vi "3- image processing.vi"() -> ()   [LabVIEW 2016]
uses:
  <vilib>/Instr/_visa.llb/VISA Configure Serial Port (Instr).vi
  <vilib>/vision/NI_Vision_Development_Module.lvlib
panel:
  out "decimal integer string 2":string
  out "decimal integer string":string
  in  "VISA resource name 4":refnum<visa-resource-name>
  out "return count 2":u32
  out "red":dbl
  out "green":dbl
  in  "VISA resource name 3":refnum<visa-resource-name>
  out "return count":u32
  out "green":bool
  out "red":bool
  out "Color Spectrum":dbl[](array[numeric]) format="%.2f"
  in  "Stop (F)":bool
  out "Image Out":T1(plugin-control)
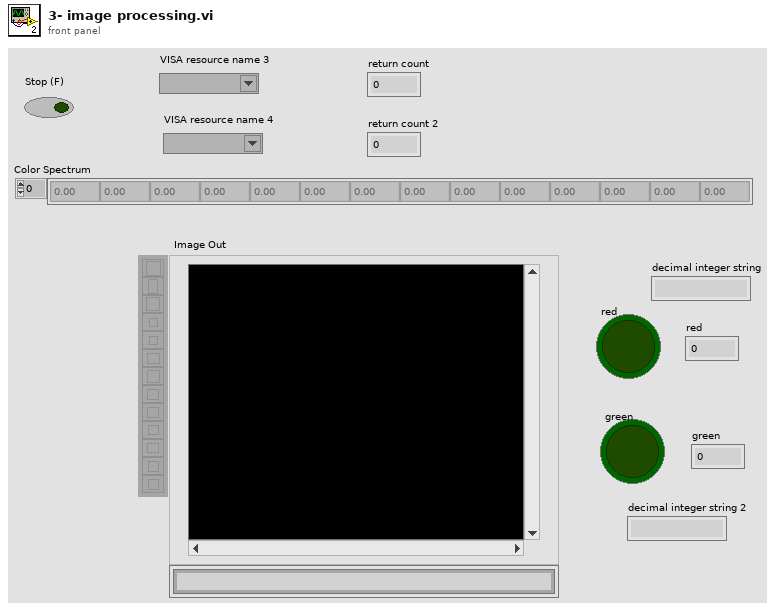
[diagram p1: front panel]
types:
  T1 = typedef "IMAQ Image.ctl" = refnum<image>
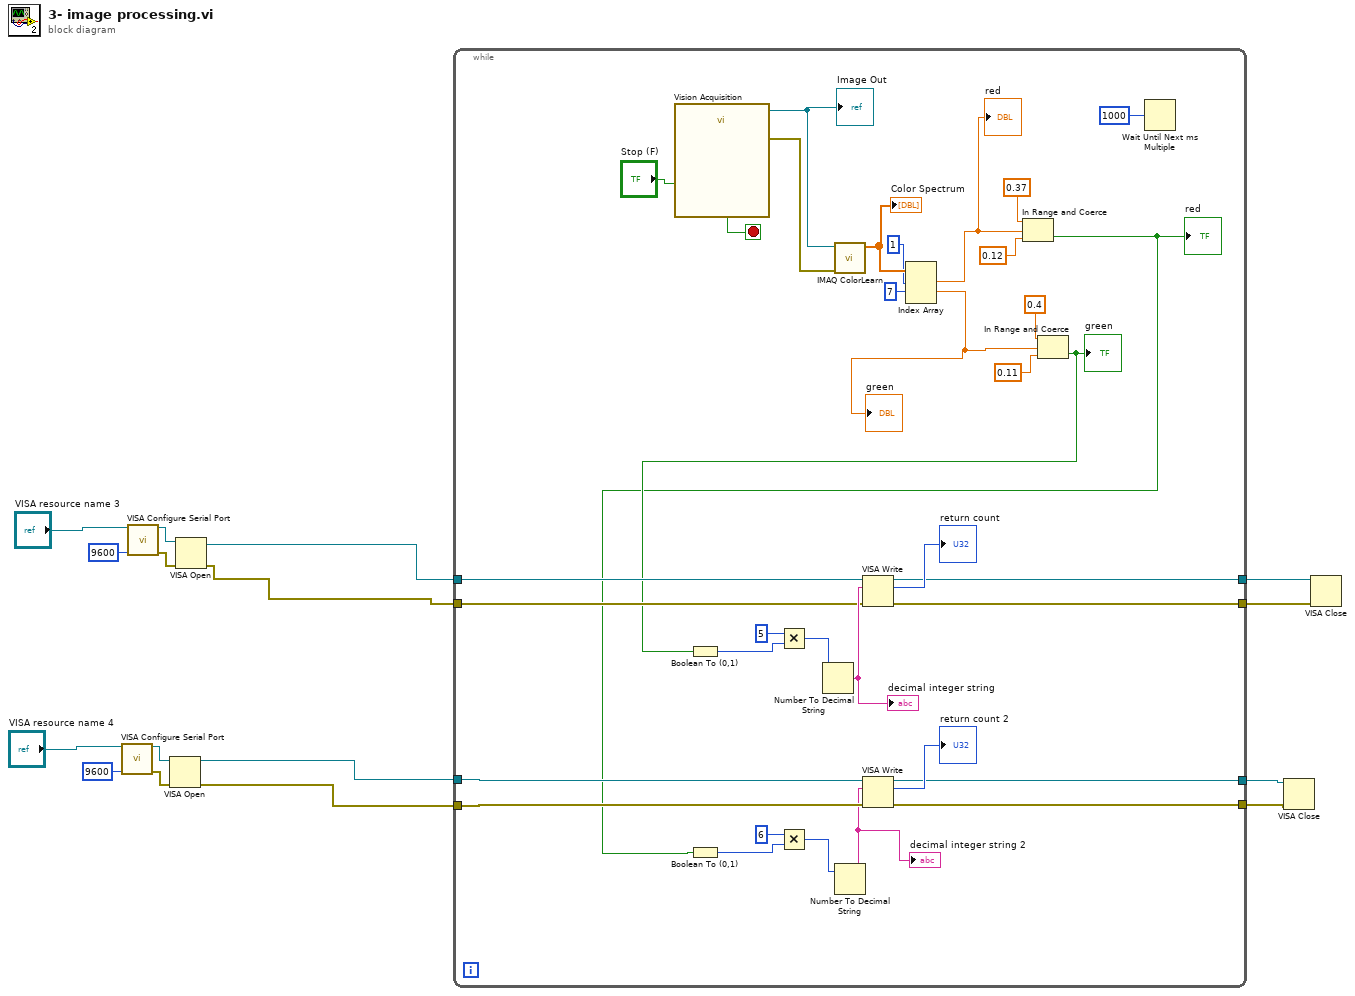
[diagram p0: block diagram]
diagram:
  n1 = call-poly "VISA Configure Serial Port"("VISA resource name"="VISA resource name 4", "baud rate (9600)"=u32 9600) -> ("VISA resource name out"=w6:refnum<visa-resource-name>, "error out"=w5:errorcluster)  [unwired: 12 in]
  n2 = call-poly "VISA Configure Serial Port"("VISA resource name"="VISA resource name 3", "baud rate (9600)"=u32 9600) -> ("VISA resource name out"=w14:refnum<visa-resource-name>, "error out"=w13:errorcluster)  [unwired: 12 in]
  n3 = VISA Open(error in (no error)=w5, VISA resource name=w6) -> (VISA resource name=w4:refnum<visa-resource-name>, error out=w3:errorcluster)  [unwired: 3 in]
  n4 = VISA Open(error in (no error)=w13, VISA resource name=w14) -> (VISA resource name=w10:refnum<visa-resource-name>, error out=w9:errorcluster)  [unwired: 3 in]
  n5 = while {
    tunnel: [w34] -> w12
    tunnel: [w33] -> w11
    tunnel: w10 -> [w32]
    tunnel: w9 -> [w31]
    tunnel: w4 -> [w23]
    tunnel: w3 -> [w22]
    tunnel: [w21] -> w2
    tunnel: [w20] -> w1
    stop <- w49 stop-if-true
    n6 = call "Vision Acquisition"("Stop (F)"="Stop (F)") -> ("Image Out"=w48:T1, "Stopped"=w49:bool, "error out"=w40:errorcluster)  [unwired: 24 in]
    "Image Out" <- w48
    n7 = call "IMAQ ColorLearn"("Image"=w48, "error in (no error)"=w40) -> ("Color Spectrum"=w47:dbl[])  [unwired: 6 in, 1 out]
    "Color Spectrum" <- w47
    n8 = Index Array(array=w47, index #1=1 ("index"), index #2=7 ("index")) -> (element #1=w18:dbl, element #2=w28:dbl)  [unwired: 1 in, 1 out]
    "green" <- w28
    "red" <- w18
    n9 = In Range and Coerce(upper limit=0.37, x=w18, lower limit=0.12) -> (In Range?=w19:bool)  [unwired: 1 out]
    "red" <- w19
    n10 = Boolean To (0,1)(Boolean=w19) -> (0, 1=w24:i16)
    n11 = Multiply(x=i16 6, y=w24) -> (x*y=w27:i16)
    n12 = Number To Decimal String(number=w27) -> (decimal integer string=w17:string)  [unwired: 1 in]
    "decimal integer string 2" <- w17
    n13 = VISA Write(VISA resource name=w23, write buffer=w17, error in (no error)=w22) -> (VISA resource name out=w21:refnum<visa-resource-name>, return count=→"return count 2":u32, error out=w20:errorcluster)
    n14 = In Range and Coerce(upper limit=0.4, x=w28, lower limit=0.11) -> (In Range?=w29:bool)  [unwired: 1 out]
    "green" <- w29
    n15 = Boolean To (0,1)(Boolean=w29) -> (0, 1=w30:i16)
    n16 = Multiply(x=i16 5, y=w30) -> (x*y=w39:i16)
    n17 = Number To Decimal String(number=w39) -> (decimal integer string=w38:string)  [unwired: 1 in]
    "decimal integer string" <- w38
    n18 = VISA Write(VISA resource name=w32, write buffer=w38, error in (no error)=w31) -> (VISA resource name out=w34:refnum<visa-resource-name>, return count=→"return count":u32, error out=w33:errorcluster)
    n19 = Wait Until Next ms Multiple(millisecond multiple=u32 1000) -> ()  [unwired: 1 out]
  }
  n20 = VISA Close(VISA resource name=w2, error in (no error)=w1) -> ()  [unwired: 1 out]
  n21 = VISA Close(VISA resource name=w12, error in (no error)=w11) -> ()  [unwired: 1 out]
